vi "ISPP Reset SL.vi"(5 "Start Voltage":dbl=1.0 format="%#_13g", 6 "Target resistance (ohm)":dbl, 7 "Step size":dbl=0.2, 8 "error in (no error)":errorcluster, 9 "SL voltage ref":refnum<vi>, 10 "WL voltage ref":refnum<vi>, 11 "instrument handle":refnum<k15>) -> (0 "error out":errorcluster, 2 "Final resistance (ohm)":dbl, 3 "instrument handle out":refnum<k15>)   [LabVIEW 2018]
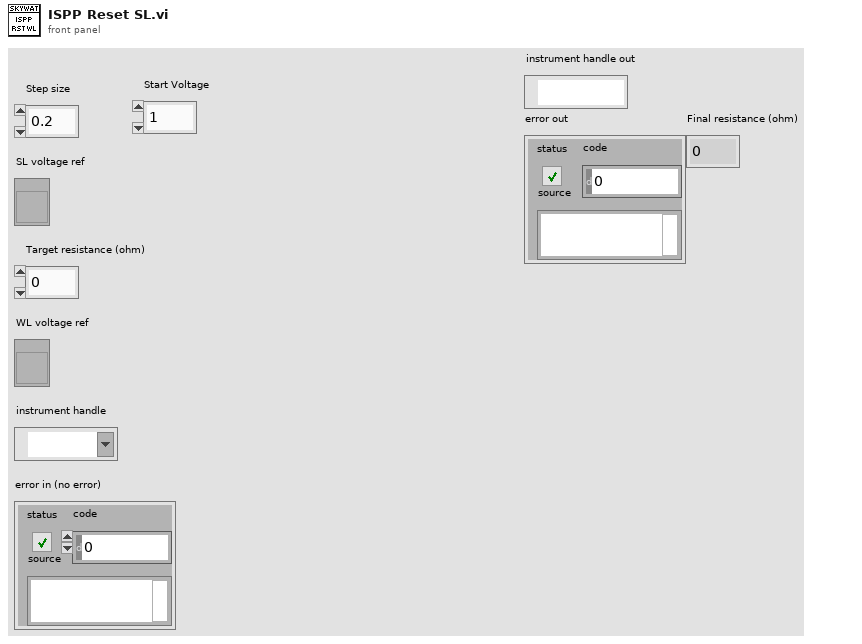
[diagram p1: front panel]
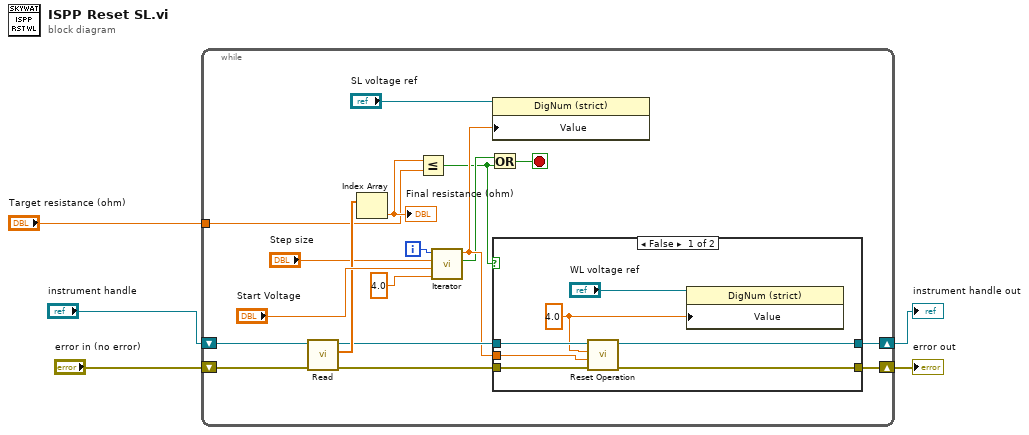
[diagram p0: block diagram]
diagram:
  n1 = while {
    shift-right: [w16] -> w2
    shift-left: "instrument handle" -> [w13]
    shift-right: [w15] -> w1
    shift-left: "error in (no error)" -> [w14]
    tunnel: "Target resistance (ohm)" -> [w8]
    i -> [w22]
    stop <- w11 stop-if-true
    n2 = call "Read.vi"("error in (no error)"=w14, "instrument handle"=w13) -> ("error out"=w19:errorcluster, "resistances (ohm)"=w20:dbl[], "instrument handle out"=w18:refnum<k15>)  [unwired: 6 in, 1 out]
    n3 = Index Array(array=w20) -> (element=w12:dbl)  [unwired: 1 in]
    "Final resistance (ohm)" <- w12
    n4 = Less Or Equal?(x=w12, y=w8) -> (x <= y?=w9:bool)
    n5 = call "Iterator.vi"("Final Value"=4.0 ("y"), "Initial Value"="Start Voltage", "Step"="Step size", "i"=w22) -> ("End Loop"=w10:bool, "Current Value"=w17:dbl)  [unwired: 6 in]
    n6 = Or(x=w10, y=w9) -> (x .or. y?=w11:bool)
    n7 = property class="DigNum (strict)"(reference="SL voltage ref", "Value"=w17) -> ()  [unwired: 1 in, 2 out]
    n8 = case shown="False" w9 {
      tunnel: [w29 w31] -> w15
      tunnel: [w30 w32] -> w16
      tunnel: w19 -> [w28 w31]
      tunnel: w18 -> [w27 w32]
      tunnel: w17 -> [w25 _]
      frame False {
        w24 = 4.0 ("level (V)")
        n9 = call "Reset Operation.vi"("error in (no error)"=w28, "SLV"=w25, "WLV"=w24, "instrument handle"=w27) -> ("error out"=w29:errorcluster, "instrument handle out"=w30:refnum<k15>)  [unwired: 6 in]
        n10 = property class="DigNum (strict)"(reference="WL voltage ref", "Value"=w24) -> ()  [unwired: 1 in, 2 out]
      }
      frame True {
      }
    }
  }
  "instrument handle out" <- w2
  "error out" <- w1
